vi "FileIO - Read-Write System Parameters.vi"(7 "Action":T2, 8 "error in (no error)":errorcluster, 11 "System Parameters in":T1={"Results FilePath"=path "", "Analysis Parameters"={"Area"={"Lower Value"=10.0, "Upper Value"=500.0}, "Circle Filter Radius"={"Lower Value"=10.0, "Upper Value"=500.0}, "Edge Detection Threshold"=50}, "ROI Parameters"={"ROI size (in Radius)"={"Width"=1.0, "Height"=0.5}}}) -> (0 "error out":errorcluster, 3 "System Parameters out":T1={"Results FilePath"=path "", "Analysis Parameters"={"Area"={"Lower Value"=10.0, "Upper Value"=500.0}, "Circle Filter Radius"={"Lower Value"=10.0, "Upper Value"=500.0}, "Edge Detection Threshold"=50}, "ROI Parameters"={"ROI size (in Radius)"={"Width"=1.0, "Height"=0.5}}})   [LabVIEW 2014]
uses:
  TypeDef - File Actions.ctl
  Custom Controls/TypeDef - System Configuration.ctl
  TypeDef - Directory Structures.ctl
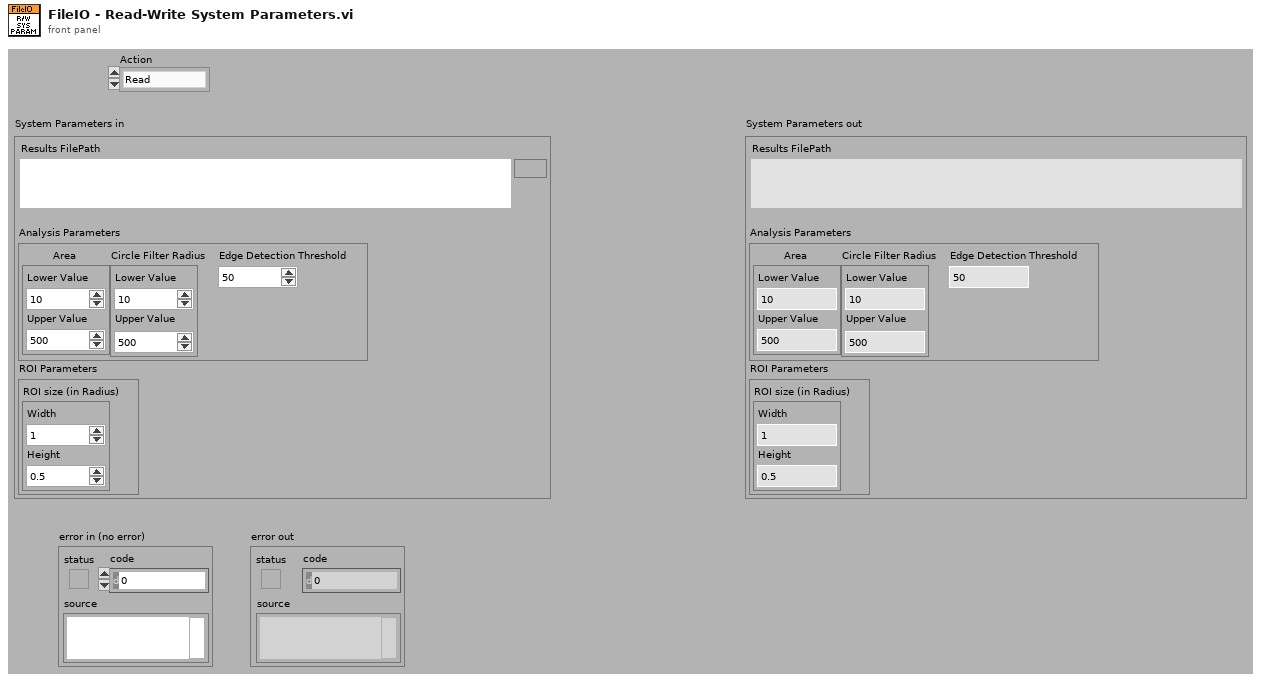
[diagram p1: front panel]
types:
  T1 = typedef "TypeDef - System Configuration.ctl" = cluster{"Results FilePath":path, "Analysis Parameters":cluster{"Area":cluster{"Lower Value":dbl, "Upper Value":dbl}, "Circle Filter Radius":cluster{"Lower Value":sgl, "Upper Value":sgl}, "Edge Detection Threshold":u16}, "ROI Parameters":cluster{"ROI size (in Radius)":cluster{"Width":dbl, "Height":dbl}}}
  T2 = typedef "TypeDef - File Actions.ctl" = enum16{"Read", "Write", "Get Current"}
  T3 = typedef "TypeDef - Directory Structures.ctl" = enum16{"Project", "config", "testconfig", "raw data"}
  T4 = enum16{"open", "replace", "create", "open or create", "replace or create", "replace or create with confirmation"}
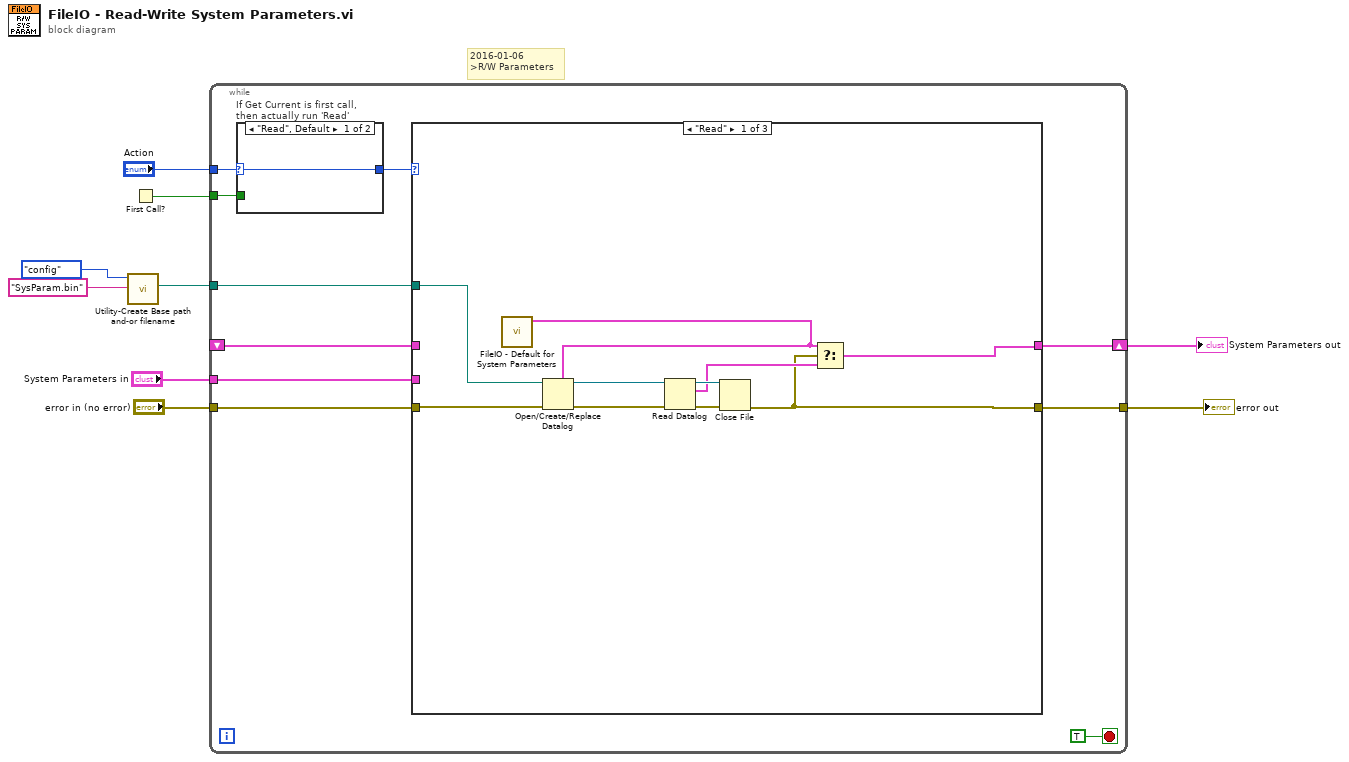
[diagram p0: block diagram]
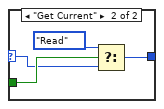
[diagram p2: hidden frame]
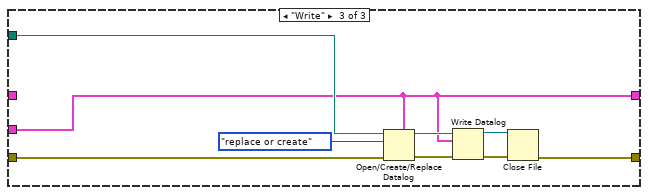
[diagram p4: hidden frame]
diagram:
  # "2016-01-06\n>R/W Parameters"
  n1 = call "Utility-Create Base path and-or filename.vi"("filename"="SysParam.bin", "Directory Name"=TypeDef_-_Directory_Structures."config") -> ("File name and path"=w6:path)  [unwired: 9 in]
  n2 = First Call?() -> (First Call?: T/F=w2:bool)
  n3 = while {
    tunnel: "error in (no error)" -> [w19]
    tunnel: [w18] -> w8
    tunnel: w6 -> [w16]
    shift-right: [w15] -> w4
    shift-left: _ -> [w17]
    tunnel: "Action" -> [w13]
    tunnel: w2 -> [w11]
    tunnel: "System Parameters in" -> [w10]
    stop <- TRUE stop-if-true
    n4 = case "If Get Current is first call, \nthen actually run 'Read'" shown="\"Read\", Default" w13 {
      selector: w13 -> [w20 w23]
      tunnel: [w20 w22] -> w12
      tunnel: w11 -> [_ w24]
      frame "Read", Default {
      }
      frame "Get Current" {
        n5 = Select(t=TypeDef_-_File_Actions."Read", s=w24, f=w23) -> (s? t:f=w22:T2)
      }
    }
    n6 = case shown="\"Read\"" w12 {
      tunnel: w17 -> [_ w35 _]
      tunnel: [w26 w35 w37] -> w15
      tunnel: w19 -> [w30 w36 w41]
      tunnel: [w27 w36 w40] -> w18
      tunnel: w16 -> [w29 _ w38]
      tunnel: w10 -> [_ _ w37]
      frame "Read" {
        n7 = call "FileIO - Default for System Parameters.vi"() -> ("Sys Parameters"=w25:T1)  [unwired: 11 in]
        n8 = Open/Create/Replace Datalog(5:w25, 8:w30, 11:w29) -> (0:w33:errorcluster, 3:w34:refnum<k1>)  [unwired: 4 out]
        n9 = Read Datalog(4:w33, 7:w34) -> (0:w32:errorcluster, 2:w28:T1, 3:w31:refnum<k1>)  [unwired: 1 out]
        n10 = Close File(refnum=w31, error in=w32) -> (error out=w27:errorcluster)  [unwired: 1 out]
        n11 = Select(t=w25, s=w27, f=w28) -> (s? t:f=w26:T1)
      }
      frame "Get Current" {
      }
      frame "Write" {
        n12 = Open/Create/Replace Datalog(5:w37, 8:w41, 10:T4."replace or create" ("operation (0:open)"), 11:w38) -> (0:w42:errorcluster, 3:w43:refnum<k1>)  [unwired: 3 out]
        n13 = Write Datalog(4:w42, 6:w37, 7:w43) -> (0:w45:errorcluster, 3:w44:refnum<k1>)
        n14 = Close File(refnum=w44, error in=w45) -> (error out=w40:errorcluster)  [unwired: 1 out]
      }
    }
  }
  "error out" <- w8
  "System Parameters out" <- w4
